vi "sensors and variables.vi"(11 "S P & V definitions":T1[](array[typedef]) {"value" format="%#_6p"; "variable"."Data average interval" min=0.0 format="%^#_3g"}) -> (0 "name (unit)":string[](array[string]), 1 "units":string[](array[string]), 2 "Variable names":string[](array[string]), 3 "Variable values":dbl[](array[numeric]))   [LabVIEW 2012]
uses:
  variable setpoint.ctl
  data ave interval.ctl
  type specifier for control code.ctl
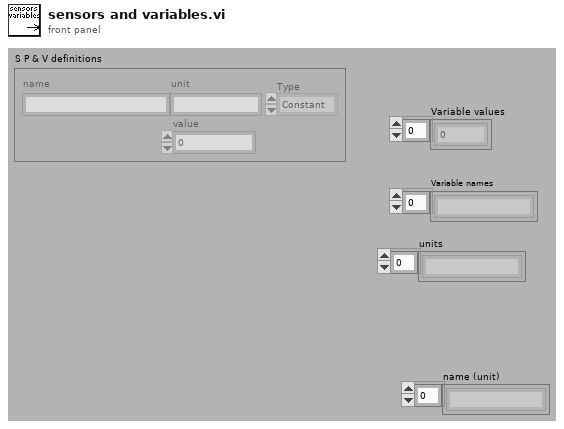
[diagram p1: front panel]
types:
  T1 = typedef "variable setpoint.ctl" = cluster{"name":string, "unit":string, "value":dbl, "Type":enum16{"Constant", "Variable"}, "variable":cluster{"selected sensors":i32[], "selected set points":i32[], "VI":path, "Data average interval":T2, "code ref":T3}}
  T2 = typedef "data ave interval.ctl" = dbl
  T3 = typedef "type specifier for control code.ctl" = refnum<vi>
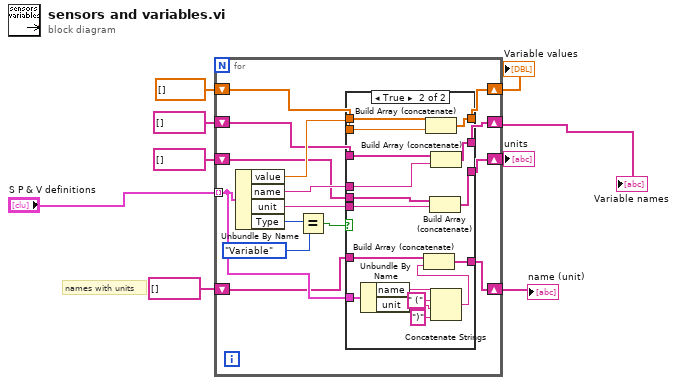
[diagram p0: block diagram]
diagram:
  # "names with units"
  n1 = for {
    tunnel: "S P & V definitions" -> [w12] mode=indexing
    shift-right: [w21] -> w5
    shift-left: string[] [] -> [w14]
    shift-right: [w18] -> w6
    shift-left: dbl[] [] -> [w19]
    shift-right: [w15] -> w3
    shift-left: string[] [] -> [w13]
    shift-right: [w10] -> w1
    shift-left: string[] [] -> [w11]
    n2 = Unbundle By Name(w12) -> ("value"=w20:dbl, "name"=w22:string, "unit"=w16:string, "Type"=w17:enum16{"Constant", "Variable"})
    n3 = Equal?(x=w17, y=enum16{"Constant", "Variable"}."Variable" ("Type")) -> (x = y?=w23:bool)
    n4 = case shown="True" w23 {
      tunnel: w22 -> [_ w40]
      tunnel: w14 -> [w28 w45]
      tunnel: [w28 w44] -> w21
      tunnel: w20 -> [_ w43]
      tunnel: w19 -> [w27 w42]
      tunnel: [w27 w41] -> w18
      tunnel: w16 -> [_ w39]
      tunnel: [w26 w38] -> w15
      tunnel: w13 -> [w26 w37]
      tunnel: w12 -> [_ w33]
      tunnel: w11 -> [w25 w30]
      tunnel: [w25 w29] -> w10
      frame False {
      }
      frame True {
        n5 = Unbundle By Name(w33) -> ("name"=w32:string, "unit"=w35:string)
        n6 = Build Array (concatenate)(w42, w43) -> (w41:dbl[])
        n7 = Build Array (concatenate)(w37, w39) -> (w38:string[])
        n8 = Build Array (concatenate)(w45, w40) -> (w44:string[])
        n9 = Concatenate Strings(w32, " (" ("string"), w35, ")" ("string")) -> (w31:string)
        n10 = Build Array (concatenate)(w30, w31) -> (w29:string[])
      }
    }
  }
  "Variable names" <- w5
  "Variable values" <- w6
  "units" <- w3
  "name (unit)" <- w1
